vi "HHMI - Generate File paths.vi"(8 "error in":errorcluster) -> (0 "error out":errorcluster, 1 "Project path":path, 2 ".ini path":path)   [LabVIEW 2013]
doc: "This .vi generates the base path, .ini paths, and dynamically called .vi's based off of the project file (project file searched for) and sets these in a filepath global. The dynamically called .vi's are checked that they exist.\n\nThis subvi can also be used in other top level Quartz apps. It only runs on first call, so it can be safely repeatedly called, in any vi within the project."
uses:
  HHMI - Filepaths global.vi
panel:
  out "Sim path":path
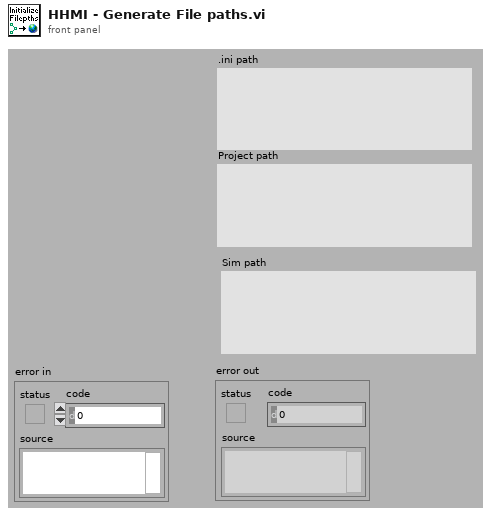
[diagram p1: front panel]
types:
  T1 = typedef "ProjectName enum.ctl" = enum16{"V-SIM", "SPIM", "TEMca2", "undefined", "HHMI Panels", "Wing Beat Analyzer"}
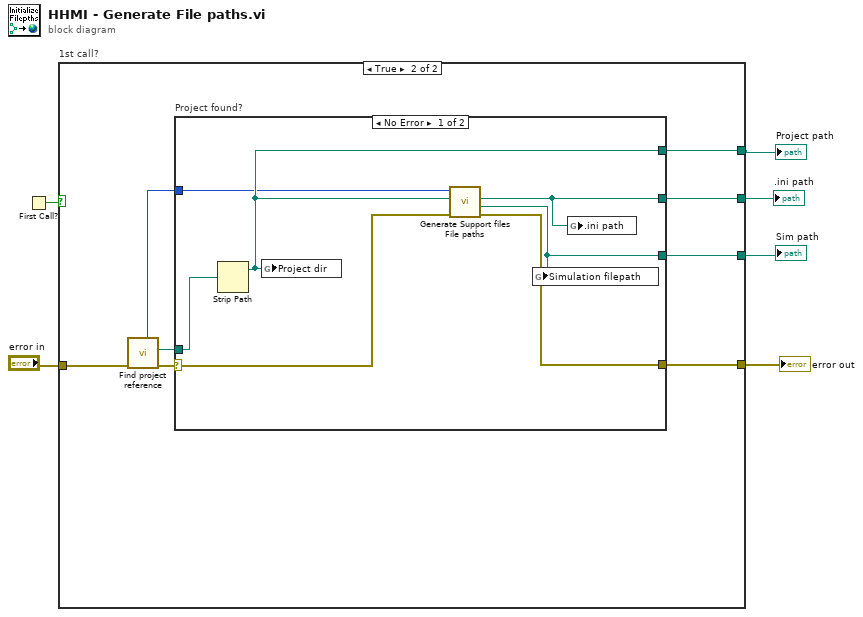
[diagram p0: block diagram]
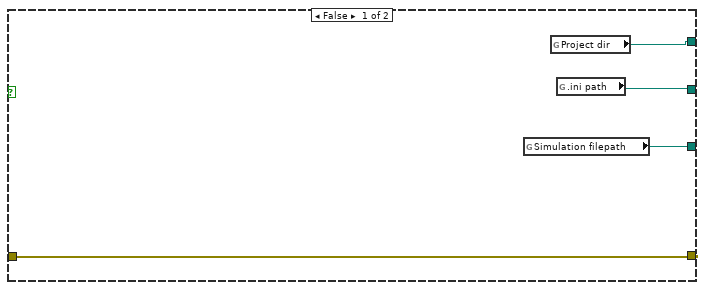
[diagram p2: hidden frame]
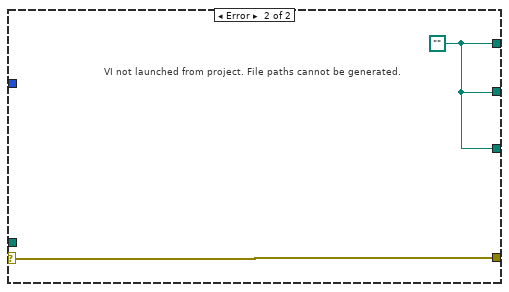
[diagram p3: hidden frame]
diagram:
  n1 = First Call?() -> (First Call?: T/F=w4:bool)
  n2 = case "1st call?" shown="True" w4 {
    tunnel: [w10 w12] -> w6
    tunnel: "error in" -> [w10 w15]
    tunnel: [w9 w13] -> w3
    tunnel: [w8 w14] -> w2
    tunnel: [w7 w11] -> w1
    frame False {
      n3 = global read "HHMI - Filepaths global.vi" "Simulation filepath"() -> (w7:path)
      n4 = global read "HHMI - Filepaths global.vi" "Project dir"() -> (w8:path)
      n5 = global read "HHMI - Filepaths global.vi" ".ini path"() -> (w9:path)
    }
    frame True {
      n6 = call "Find project reference.vi"("error in"=w15) -> ("ProjectName"=w17:T1, ".lvproj Filepath"=w18:path, "error out"=w16:errorcluster)  [unwired: 5 out]
      n7 = case "Project found?" shown="No Error" w16 {
        selector: w16 -> [w21 w27]
        tunnel: w18 -> [w25 _]
        tunnel: [w23 w27] -> w12
        tunnel: [w20 w26] -> w13
        tunnel: [w24 w26] -> w14
        tunnel: w17 -> [w22 _]
        tunnel: [w19 w26] -> w11
        frame No Error {
          n8 = Strip Path(path=w25) -> (stripped path=w24:path)  [unwired: 1 out]
          n9 = global write "HHMI - Filepaths global.vi" "Project dir"(w24) -> ()
          n10 = call "Generate Support files File paths.vi"("error in"=w21, "base path"=w24, "ProjectName"=w22) -> ("error out"=w23:errorcluster, "Log path"=w19:path, ".ini path"=w20:path)  [unwired: 2 out]
          n11 = global write "HHMI - Filepaths global.vi" "Simulation filepath"(w19) -> ()
          n12 = global write "HHMI - Filepaths global.vi" ".ini path"(w20) -> ()
        }
        frame Error {
          w26 = path ""
          # "VI not launched from project. File paths cannot be generated."
        }
      }
    }
  }
  "error out" <- w6
  ".ini path" <- w3
  "Project path" <- w2
  "Sim path" <- w1
